vi "new exception.vi"(11 "context":T2) -> (1 "exception":T1 {"code" format="%.0x"})   [LabVIEW 2013, in "exception.lvlib"]
uses:
  exception.lvlib
  context.ctl
  exception.ctl
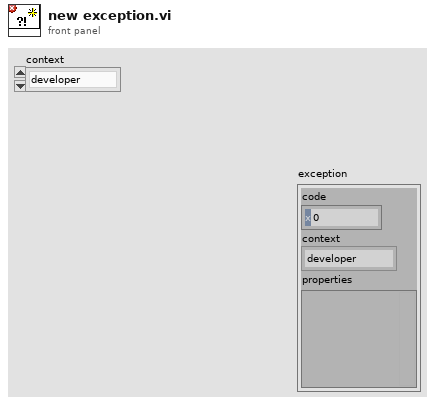
[diagram p1: front panel]
types:
  T1 = typedef "exception.lvlib/exception.ctl" = cluster{"code":i32, "context":T2, "properties":variant}
  T2 = typedef "exception.lvlib/context.ctl" = enum16{"developer", "user interface", "standard", "limited", "deterministic"}
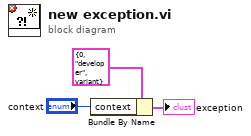
[diagram p0: block diagram]
diagram:
  n1 = Bundle By Name(cluster=T1 {"code"=0, "context"=enum."developer", "properties"=variant} ("exception"), "context"="context") -> (→"exception":T1)
